vi "data check.vi"() -> ()   [LabVIEW 2020]
panel:
  out "element 8":u64 format="%.0x"
  out "element 7":u64 format="%.0x"
  out "element 6":u64 format="%.0x"
  out "element 5":u64 format="%.0x"
  out "element 4":u32 format="%.0x"
  out "element 3":u64 format="%.0x"
  out "element 2":u64 format="%.0x"
  out "element":u64 format="%.0x"
  out "Array":u64[](array[numeric]) format="%.0x"
  in  "Array 2":u64[](array[numeric]) format="%.0x"
  out "max(x,y)":i32[](array[numeric])
  out "x*y":i32
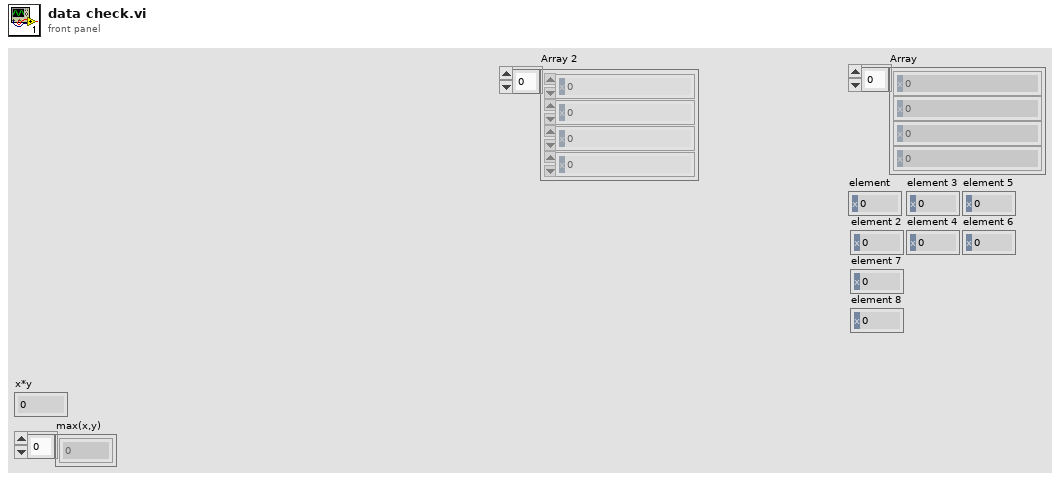
[diagram p1: front panel]
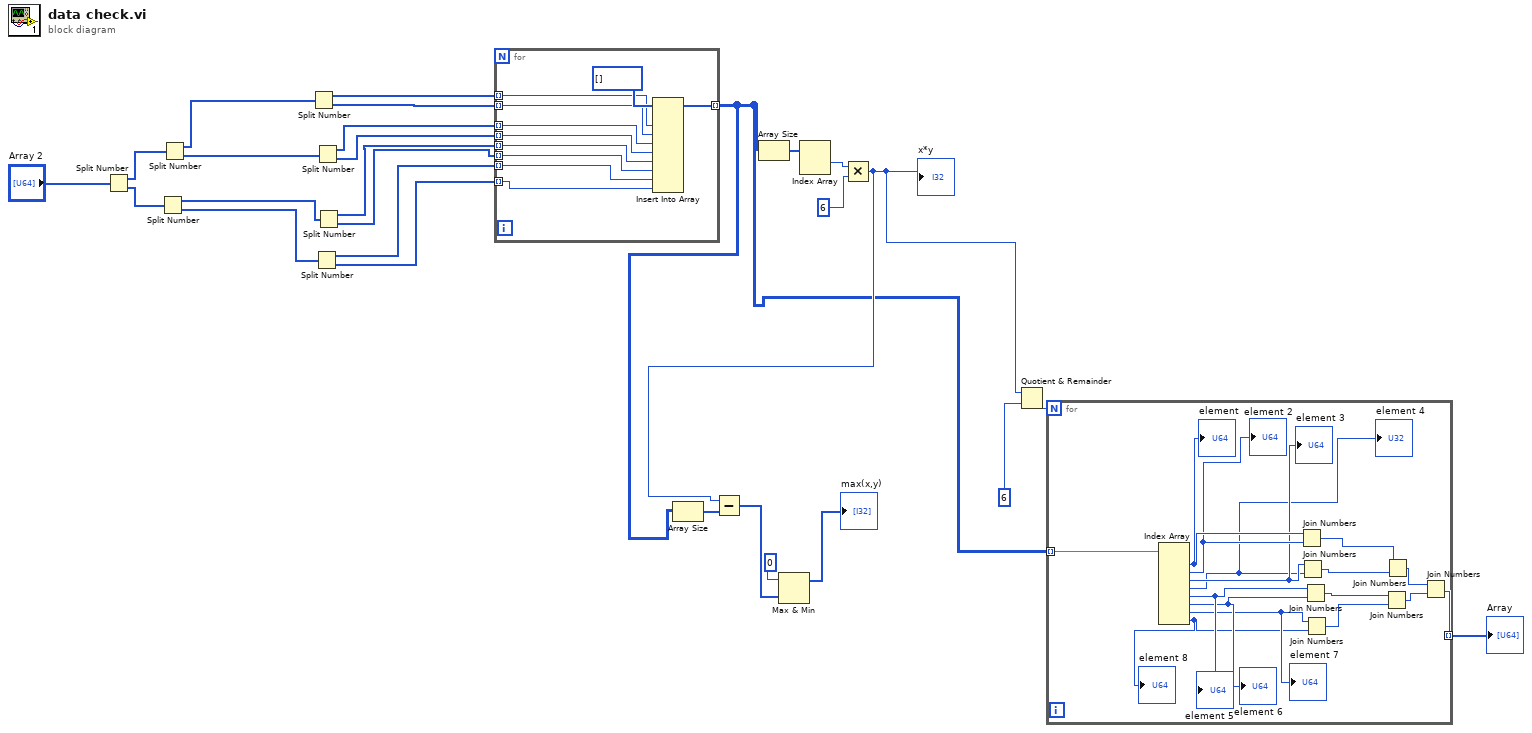
[diagram p0: block diagram]
diagram:
  n1 = Split Number(x="Array 2") -> (hi(x)=w15:u32[], lo(x)=w14:u32[])
  n2 = Split Number(x=w14) -> (hi(x)=w9:u16[], lo(x)=w8:u16[])
  n3 = Split Number(x=w15) -> (hi(x)=w13:u16[], lo(x)=w12:u16[])
  n4 = Split Number(x=w13) -> (hi(x)=w2:u8[], lo(x)=w1:u8[])
  n5 = Split Number(x=w8) -> (hi(x)=w5:u8[], lo(x)=w4:u8[])
  n6 = Split Number(x=w12) -> (hi(x)=w11:u8[], lo(x)=w10:u8[])
  n7 = Split Number(x=w9) -> (hi(x)=w7:u8[], lo(x)=w6:u8[])
  n8 = for {
    tunnel: [w37] -> w17 mode=indexing
    tunnel: w11 -> [w33] mode=indexing
    tunnel: w10 -> [w32] mode=indexing
    tunnel: w7 -> [w31] mode=indexing
    tunnel: w6 -> [w30] mode=indexing
    tunnel: w5 -> [w29] mode=indexing
    tunnel: w4 -> [w28] mode=indexing
    tunnel: w2 -> [w35] mode=indexing
    tunnel: w1 -> [w34] mode=indexing
    n9 = Insert Into Array(array=u8[] [], new element #1=w35, new element #2=w34, new element #3=w33, new element #4=w32, new element #5=w31, new element #6=w30, new element #7=w29, new element #8=w28) -> (w37:u8[])  [unwired: 1 in]
  }
  n10 = Array Size(array=w17) -> (size(s)=w22:i32[])
  n11 = Array Size(array=w17) -> (size(s)=w27:i32[])
  n12 = Index Array(array=w27) -> (element #1=w21:i32)  [unwired: 2 in, 1 out]
  n13 = Multiply(x=w21, y=6) -> (x*y=w18:i32)
  "x*y" <- w18
  n14 = Subtract(x=w18, y=w22) -> (x-y=w25:i32[])
  n15 = Max & Min(x=0, y=w25) -> (max(x,y)=→"max(x,y)":i32[])  [unwired: 1 out]
  n16 = Quotient & Remainder(x=w18, y=6) -> (floor(x/y)=w19:i32)  [unwired: 1 out]
  n17 = for {
    N: w19 -> [_]
    tunnel: [w53] -> w3 mode=indexing
    tunnel: w17 -> [w52] mode=indexing
    n18 = Index Array(array=w52) -> (element #1=w45:u8, element #2=w44:u8, element #3=w43:u8, element #4=w42:u8, element #5=w41:u8, element #6=w40:u8, element #7=w39:u8, element #8=w38:u8)  [unwired: 8 in]
    "element 5" <- w41
    "element 6" <- w40
    "element 7" <- w39
    "element 8" <- w38
    "element" <- w45
    "element 2" <- w44
    "element 3" <- w43
    "element 4" <- w42
    n19 = Join Numbers(hi=w45, lo=w44) -> ((hi.lo)=w47:u16)
    n20 = Join Numbers(hi=w43, lo=w42) -> ((hi.lo)=w46:u16)
    n21 = Join Numbers(hi=w41, lo=w40) -> ((hi.lo)=w49:u16)
    n22 = Join Numbers(hi=w39, lo=w38) -> ((hi.lo)=w48:u16)
    n23 = Join Numbers(hi=w49, lo=w48) -> ((hi.lo)=w50:u32)
    n24 = Join Numbers(hi=w47, lo=w46) -> ((hi.lo)=w51:u32)
    n25 = Join Numbers(hi=w51, lo=w50) -> ((hi.lo)=w53:u64)
  }
  "Array" <- w3
